vi "Create Option.vi"(8 "error in (no error)":errorcluster, 11 "Option Config":T1) -> (0 "error out":errorcluster, 3 "Option out":refnum<class "Option.lvclass">)   [LabVIEW 2011, in "Option Parser.lvlib" / "Option.lvclass"]
uses:
  Option.lvclass
  Option Configuration.ctl
  Argument Type.ctl
  Option.lvclass/Option.ctl
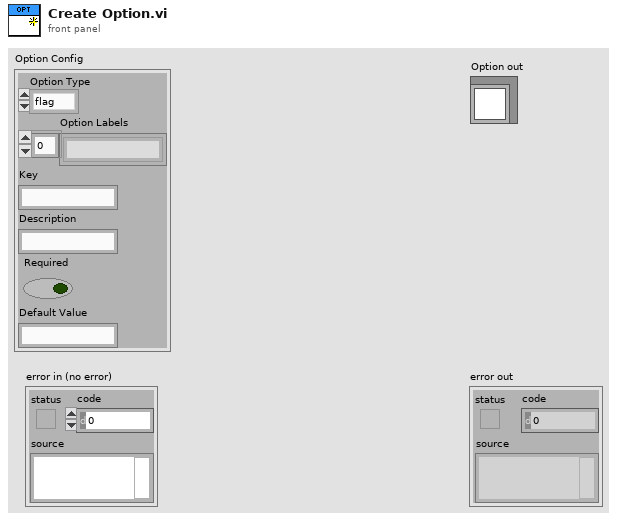
[diagram p1: front panel]
types:
  T1 = typedef "Option Parser.lvlib/Option.lvclass/Option Configuration.ctl" = cluster{"Option Type":T2, "Option Labels":string[], "Key":string, "Description":string, "Required":bool, "Default Value":string}
  T2 = typedef "Option Parser.lvlib/Option.lvclass/Argument Type.ctl" = enum16{"flag", "value"}
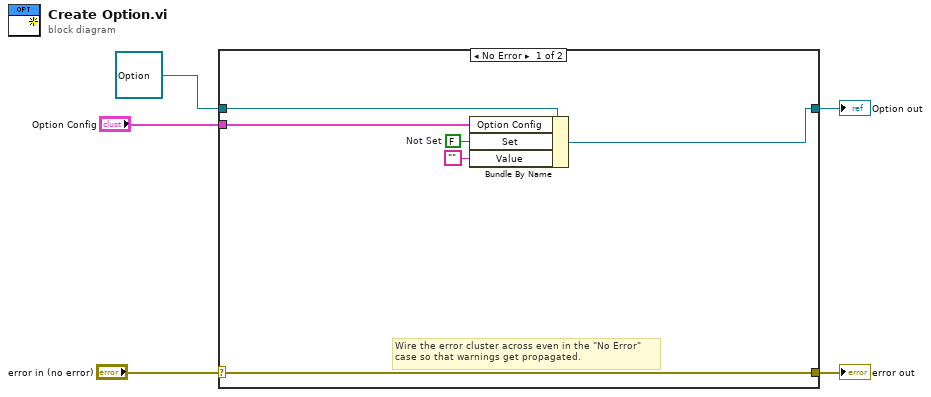
[diagram p0: block diagram]
diagram:
  n1 = case shown="No Error" "error in (no error)" {
    selector: "error in (no error)" -> [w10 w13]
    tunnel: [w10 w13] -> w4
    tunnel: [w9 w12] -> w3
    tunnel: refnum<class "Option.lvclass"> refnum ("Option in") -> [w11 w12]
    tunnel: "Option Config" -> [w8 _]
    frame No Error {
      w7 = FALSE  # Not Set
      # "Wire the error cluster across even in the \"No Error\"\ncase so that warnings get propagated."
      n2 = Bundle By Name(cluster=w11, "Option Config"=w8, "Set"=w7, "Value"="") -> (w9:refnum<class "Option.lvclass">)
    }
    frame Error {
    }
  }
  "error out" <- w4
  "Option out" <- w3
